vi "IrMainBootstrap.vi"() -> ()   [LabVIEW 2017]
uses:
  <vilib>/NI/Software Watchdog/Pound/Pound.lvclass
  <vilib>/addons/BlinkProcess/controls/mode.ctl
  <vilib>/addons/InsightCM/Devices/Shared/Common/Controller/controls/operations.ctl
  <vilib>/addons/TraceLogger/TraceLogger.lvlib
  <vilib>/addons/Qbus/Qbus.lvclass
  <vilib>/addons/InsightCM/Devices/Shared/Common/ServerComm/ServerComm.lvlib
  <vilib>/addons/TimerProcess/TimerProcess.lvlib
  <vilib>/addons/BlinkProcess/BlinkProcess.lvlib
  <vilib>/addons/InsightCM/Devices/Shared/Common/TracePointDisplay/TracePointDisplay.lvlib
  <vilib>/addons/InsightCM/Devices/Shared/Common/Controller/Controller.lvlib
  <vilib>/addons/InsightCM/Utilities/GlobalConfiguration/GlobalConfiguration.lvlib
  <vilib>/addons/InsightCM/Devices/Shared/Ir/IrAcquisition/IrAcquisition.lvlib
  <vilib>/addons/InsightCM/Devices/Shared/Ir/IrManageCameras/IrManageCameras.lvlib
panel:
  out "Log":string
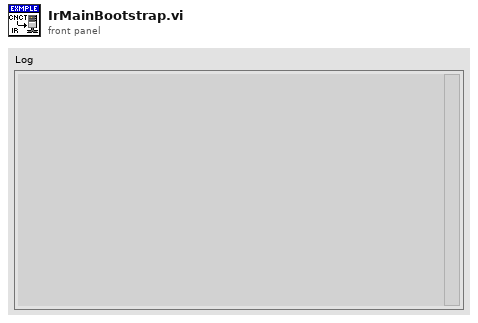
[diagram p1: front panel]
types:
  T1 = typedef "BlinkProcess.lvlib/mode.ctl" = enum16{"Normal", "Error", "On", "Off", "Custom"}
  T2 = typedef "Controller.lvlib/operations.ctl" = enum16{"Unknown", "Startup", "Expected Shutdown"}
  T3 = typedef "ServerComm.lvlib/ConnectionStatus.ctl" = enum16{"Offline", "NotAuthorized", "Online"}
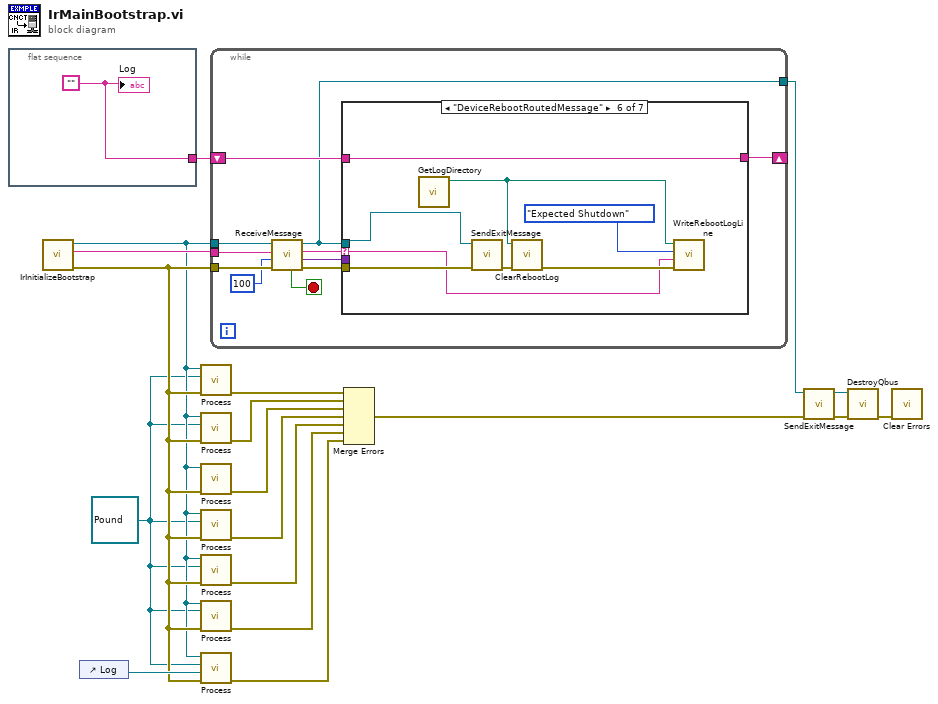
[diagram p0: block diagram]
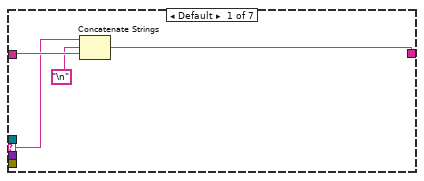
[diagram p2: hidden frame]
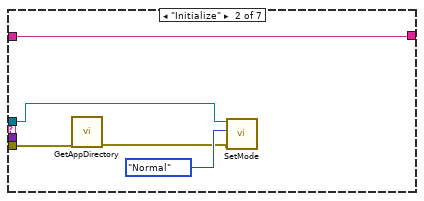
[diagram p3: hidden frame]
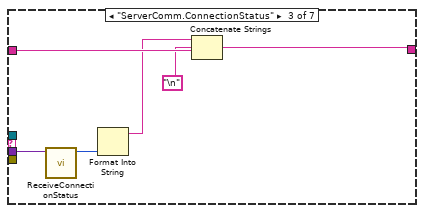
[diagram p4: hidden frame]
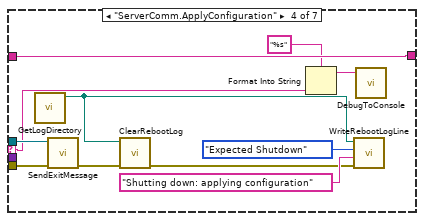
[diagram p5: hidden frame]
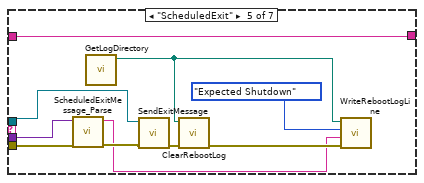
[diagram p6: hidden frame]
diagram:
  w1 = refnum<class "Pound.lvclass"> refnum ("Pound in")
  n1 = flat-sequence {
    tunnel: [w18] -> w15
    frame #0 {
      w18 = ""
      "Log" <- w18
    }
  }
  n2 = call "IrInitializeBootstrap.vi"() -> ("error out"=w5:errorcluster, "ProcessName"=w9:string, "Qbus out"=w4:refnum<class "Qbus.lvclass">)  [unwired: 9 in]
  n3 = control-ref of="Log"() -> (w6:refnum<vi>)
  n4 = call <vilib>:"Process.vi"("error in (no error)"=w5, "Pound in"=w1, "Qbus in"=w4) -> ("error out"=w2:errorcluster)  [unwired: 8 in]
  n5 = call <vilib>:"Process.vi"("error in (no error)"=w5, "Pound in"=w1, "Qbus in"=w4) -> ("error out"=w3:errorcluster)  [unwired: 8 in]
  n6 = call <vilib>:"Process.vi"("error in (no error)"=w5, "qbus in"=w4) -> ("error out"=w17:errorcluster)  [unwired: 9 in]
  n7 = call <vilib>:"Process.vi"("error in (no error)"=w5, "Pound in"=w1, "Qbus in"=w4) -> ("error out"=w16:errorcluster)  [unwired: 8 in]
  n8 = call <vilib>:"Process.vi"("error in (no error)"=w5, "pound in"=w1, "qbus in"=w4) -> ("error out"=w14:errorcluster)  [unwired: 8 in]
  n9 = call <vilib>:"Process.vi"("error in (no error)"=w5, "Pound"=w1, "Qbus in"=w4) -> ("error out"=w8:errorcluster)  [unwired: 8 in]
  n10 = call <vilib>:"Process.vi"("error in (no error)"=w5, "string refnum"=w6, "Pound in"=w1, "Qbus in"=w4) -> ("error out"=w7:errorcluster)  [unwired: 7 in]
  n11 = while {
    tunnel: w4 -> [w29]
    tunnel: w9 -> [w28]
    tunnel: w5 -> [w27]
    tunnel: [w22] -> w12
    shift-right: [w20] -> _
    shift-left: w15 -> [w24]
    stop <- w19 stop-if-true
    n12 = call <vilib>:"ReceiveMessage.vi"("error in (no error)"=w27, "timeout (0)"=100, "process name"=w28, "Qbus in"=w29) -> ("error in (no error)"=w21:errorcluster, "message value"=w23:variant, "message name"=w25:string, "Qbus out"=w22:refnum<class "Qbus.lvclass">, "exit"=w19:bool)  [unwired: 2 in, 1 out]
    n13 = case shown="\"DeviceRebootRoutedMessage\"" w25 {
      selector: w25 -> [w31 _ _ w45 _ w66 _]
      tunnel: [w32 w38 w43 w51 w65 w73 w74] -> w20
      tunnel: w24 -> [w33 w38 w44 w51 w65 w73 w74]
      tunnel: w23 -> [_ _ w42 _ w58 _ _]
      tunnel: w22 -> [_ w36 _ w50 w57 w69 _]
      tunnel: w21 -> [_ w35 _ w49 w59 w67 _]
      frame Default {
        n14 = Concatenate Strings(w31, "\n", w33) -> (w32:string)
      }
      frame "Initialize" {
        n15 = call <vilib>:"GetAppDirectory.vi"("error in (no error)"=w35) -> ("error out"=w34:errorcluster)  [unwired: 9 in, 1 out]
        n16 = call <vilib>:"SetMode.vi"("error in (no error)"=w34, "mode"=mode."Normal", "Qbus in"=w36) -> ()  [unwired: 7 in, 2 out]
      }
      frame "ServerComm.ConnectionStatus" {
        n17 = call <vilib>:"ReceiveConnectionStatus.vi"("body"=w42) -> ("status"=w41:T3)  [unwired: 7 in, 3 out]
        n18 = Format Into String(w41) -> (resulting string=w40:string)  [unwired: 3 in, 1 out]
        n19 = Concatenate Strings(w40, "\n", w44) -> (w43:string)
      }
      frame "ServerComm.ApplyConfiguration" {
        n20 = call <vilib>:"GetLogDirectory.vi"() -> ("log dir"=w48:path)  [unwired: 10 in, 1 out]
        n21 = call <vilib>:"SendExitMessage.vi"("error in (no error)"=w49, "Qbus in"=w50) -> ("error in (no error)"=w53:errorcluster)  [unwired: 8 in, 1 out]
        n22 = call <vilib>:"ClearRebootLog.vi"("error in"=w53, "log path"=w48) -> ("error out"=w52:errorcluster)  [unwired: 9 in]
        n23 = Format Into String(format string="%s", w45) -> (resulting string=w46:string)  [unwired: 2 in, 1 out]
        n24 = call <vilib>:"WriteRebootLogLine.vi"("error in"=w52, "reboot log text"="Shutting down: applying configuration", "operation"=operations."Expected Shutdown", "log path"=w48) -> ()  [unwired: 6 in, 2 out]
        n25 = call <vilib>:"DebugToConsole.vi"("String"=w46) -> ()  [unwired: 10 in, 1 out]
      }
      frame "ScheduledExit" {
        n26 = call <vilib>:"ScheduledExitMessage_Parse.vi"("error in (no error)"=w59, "scheduled exit message"=w58) -> ("error out"=w61:errorcluster, "scheduled exit reason"=w60:string)  [unwired: 8 in]
        n27 = call <vilib>:"GetLogDirectory.vi"() -> ("log dir"=w56:path)  [unwired: 10 in, 1 out]
        n28 = call <vilib>:"SendExitMessage.vi"("error in (no error)"=w61, "Qbus in"=w57) -> ("error in (no error)"=w63:errorcluster)  [unwired: 8 in, 1 out]
        n29 = call <vilib>:"ClearRebootLog.vi"("error in"=w63, "log path"=w56) -> ("error out"=w62:errorcluster)  [unwired: 9 in]
        n30 = call <vilib>:"WriteRebootLogLine.vi"("error in"=w62, "reboot log text"=w60, "operation"=operations."Expected Shutdown", "log path"=w56) -> ()  [unwired: 6 in, 2 out]
      }
      frame "DeviceRebootRoutedMessage" {
        n31 = call <vilib>:"GetLogDirectory.vi"() -> ("log dir"=w68:path)  [unwired: 10 in, 1 out]
        n32 = call <vilib>:"SendExitMessage.vi"("error in (no error)"=w67, "Qbus in"=w69) -> ("error in (no error)"=w71:errorcluster)  [unwired: 8 in, 1 out]
        n33 = call <vilib>:"ClearRebootLog.vi"("error in"=w71, "log path"=w68) -> ("error out"=w70:errorcluster)  [unwired: 9 in]
        n34 = call <vilib>:"WriteRebootLogLine.vi"("error in"=w70, "reboot log text"=w66, "operation"=operations."Expected Shutdown", "log path"=w68) -> ()  [unwired: 6 in, 2 out]
      }
      frame "" {
      }
    }
  }
  n35 = Merge Errors(w2, w3, w17, w16, w14, w8, w7) -> (w11:errorcluster)
  n36 = call <vilib>:"SendExitMessage.vi"("error in (no error)"=w11, "Qbus in"=w12) -> ("error in (no error)"=w13:errorcluster, "Qbus out"=w10:refnum<class "Qbus.lvclass">)  [unwired: 8 in]
  n37 = call <vilib>:"DestroyQbus.vi"("Qbus"=w10) -> ()  [unwired: 10 in, 1 out]
  n38 = call <vilib>:"Clear Errors.vi"("error in (no error)"=w13) -> ()  [unwired: 5 in, 2 out]
